vi "Adv占空比测量备份.vi"(0 "通道":enum16{"T1", "T2", "P", "S"}(ring), 3 "error in (no error)":errorcluster) -> (7 "占空比1":dbl, 8 "占空比2":dbl, 10 "error out":errorcluster)   [LabVIEW 2020]
uses:
  <userlib>/DAQNavi Polymorphic VI/create/DAQNavi Create Channel(CI-PulseWidth).vi
  <userlib>/DAQNavi Polymorphic VI/read/DAQNavi Read (Counter 1D Pulse Width 1Chan NSamp).vi
  <userlib>/_MGI/1D Array/MGI Average/MGI Average (DBL[]).vi
  b87dcc83-9005-4041-b36d-e98345b9a8df.vi
  c5b0fe3e-6a74-4c4c-8d09-469e5175c7ec.vi
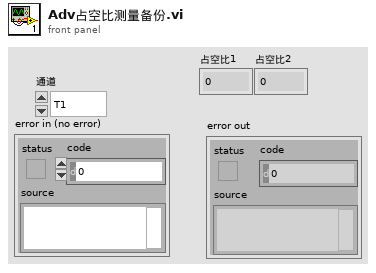
[diagram p1: front panel]
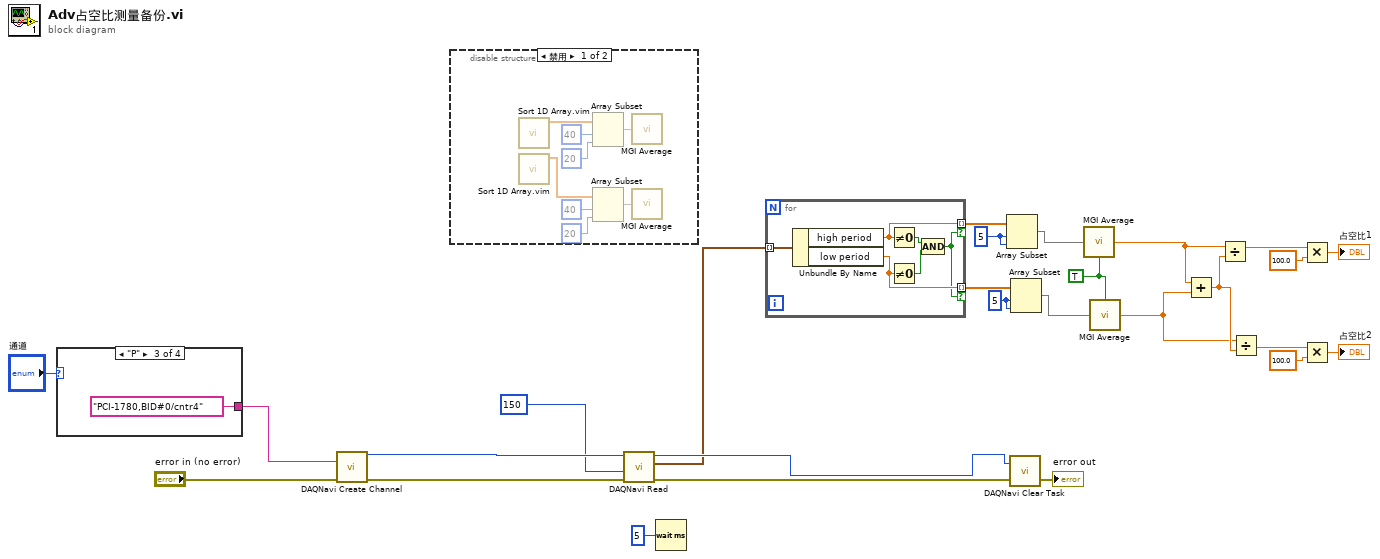
[diagram p0: block diagram]
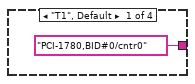
[diagram p3: hidden frame]
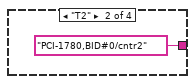
[diagram p4: hidden frame]
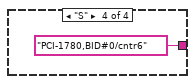
[diagram p5: hidden frame]
diagram:
  w2 = TRUE ("Ignore NaN? (F)")
  w7 = 5 ("索引")
  w8 = 5 ("索引")
  n1 = case shown="\"P\"" "通道" {
    tunnel: ["PCI-1780,BID#0/cntr0" ("physical channels") "PCI-1780,BID#0/cntr2" ("physical channels") "PCI-1780,BID#0/cntr4" ("physical channels") "PCI-1780,BID#0/cntr6" ("physical channels")] -> w27
    frame "T1", Default {
    }
    frame "T2" {
    }
    frame "P" {
    }
    frame "S" {
    }
  }
  n2 = call-poly <userlib>:"DAQNavi Create Channel.vi"("physical channels"=w27, "error in (no error)"="error in (no error)") -> ("task out"=w23:i32, "error out"=w26:errorcluster)  [unwired: 12 in]
  n3 = disable-structure shown="禁用" {
    frame Disabled {
      n4 = call "Sort 1D Array.vim"() -> ("sorted array"=w39:dbl[])  [unwired: 11 in]
      n5 = call "Sort 1D Array.vim"() -> ("sorted array"=w35:dbl[])  [unwired: 11 in]
      n6 = Array Subset(array=w39, index=40 ("索引"), length=20 ("长度")) -> (w38:dbl[])
      n7 = Array Subset(array=w35, index=40 ("索引"), length=20 ("长度")) -> (w34:dbl[])
      n8 = call-poly <userlib>:"MGI Average.vi"("Double[]"=w38) -> ()  [unwired: 1 in, 1 out]
      n9 = call-poly <userlib>:"MGI Average.vi"("Double[]"=w34) -> ()  [unwired: 1 in, 1 out]
    }
    frame Enabled {
    }
  }
  n10 = call-poly <userlib>:"DAQNavi Read.vi"("error in (no error)"=w26, "number of samples per channel to read"=u32 150, "task in"=w23) -> ("error out"=w25:errorcluster, "data"=w9:cluster{"high period":dbl, "low period":dbl}[], "task out"=w24:i32)  [unwired: 6 in]
  n11 = Wait (ms)(milliseconds to wait=u32 5 ("等待时间（毫秒）")) -> ()  [unwired: 1 out]
  n12 = for {
    tunnel: [w45] -> w14 mode=indexing if=w40
    tunnel: [w44] -> w13 mode=indexing if=w40
    tunnel: w9 -> [w41] mode=indexing
    n13 = Unbundle By Name(w41) -> ("high period"=w44:dbl, "low period"=w45:dbl)
    n14 = Not Equal To 0?(x=w44) -> (x != 0?=w42:bool)
    n15 = Not Equal To 0?(x=w45) -> (x != 0?=w43:bool)
    n16 = Compound Arithmetic op=AND ("复合运算")(w42, w43) -> (w40:bool)
  }
  n17 = Array Subset(array=w13, index=w8, length=w8) -> (w6:dbl[])
  n18 = call <userlib>:"DAQNavi Clear Task.vi"("error in (no error)"=w25, "task in"=w24) -> ("error out"=→"error out":errorcluster)  [unwired: 1 in]
  n19 = Array Subset(array=w14, index=w7, length=w7) -> (w4:dbl[])
  n20 = call-poly <userlib>:"MGI Average.vi"("Double[]"=w6, "Ignore NaN? (F)"=w2) -> ("Average"=w5:dbl)
  n21 = call-poly <userlib>:"MGI Average.vi"("Double[]"=w4, "Ignore NaN? (F)"=w2) -> ("Average"=w3:dbl)
  n22 = Add(x=w5, y=w3) -> (x+y=w22:dbl)
  n23 = Divide(x=w5, y=w22) -> (x/y=w21:dbl)
  n24 = Divide(x=w3, y=w22) -> (x/y=w20:dbl)
  n25 = Multiply(x=w21, y=100.0) -> (x*y=→"占空比1":dbl)
  n26 = Multiply(x=w20, y=100.0) -> (x*y=→"占空比2":dbl)
